vi "WS1050 BURN EFUSE.vi"() -> ()   [LabVIEW 2009]
panel:
  in  "READBACK":bool
  out "error out 2":errorcluster
  out "Fuse Readback":string
  in  "BIT TO BURN":string="07450F"
  in  "stop":bool
  out "VISA resource name out":refnum<visa-resource-name>
  out "error out":errorcluster
  in  "error in (no error)":errorcluster
  in  "VISA resource name":refnum<visa-resource-name>="COM1"
  in  "PUSH BUTTON \nTO START TEST":bool
  # "TEST PROCEDURE TO BURN FUSE T7\n\n1. BIT TO BURN \"ENTER 0745XX\"\n2. INCREASE VDD TO 5V \"JUMPER THE YELLOW WIRE TO 5V\"\n3. DECREASE VDD TO 3.3V THEN MOVE JUMPER TO GND\n4. COMPLETED\n5. READ BACK TO VERIFY FUSE"
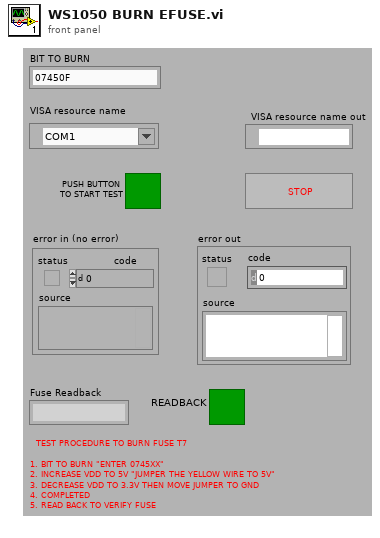
[diagram p1: front panel]
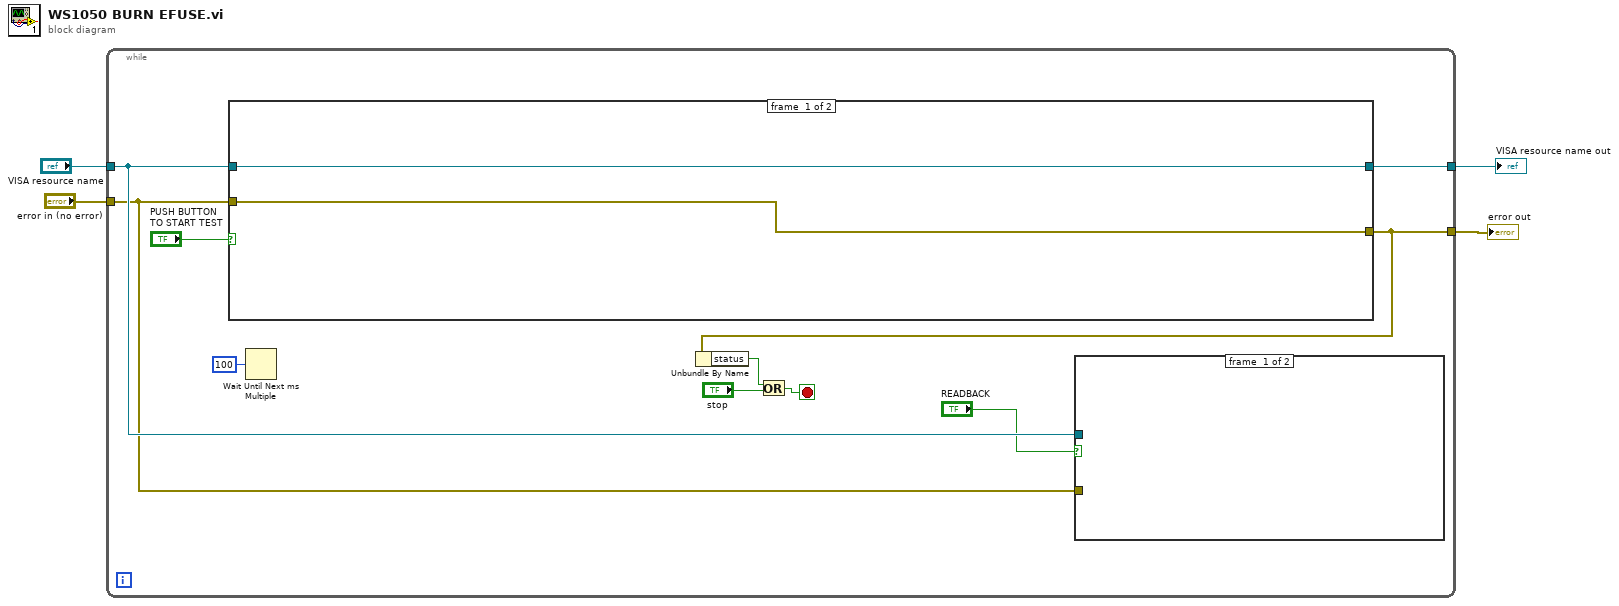
[diagram p0: block diagram]
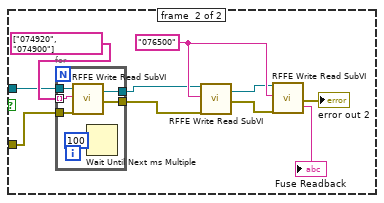
[diagram p2: hidden frame]
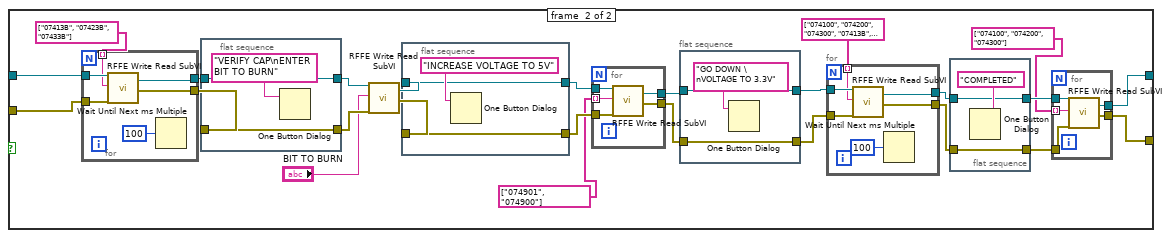
[diagram p3: hidden frame]
diagram:
  n1 = while {
    tunnel: "VISA resource name" -> [w7]
    tunnel: "error in (no error)" -> [w6]
    tunnel: [w11] -> w1
    tunnel: [w13] -> w2
    stop <- w8 stop-if-true
    n2 = case shown="True" "PUSH BUTTON \nTO START TEST" {
      tunnel: w7 -> [w31 w57]
      tunnel: w6 -> [w32 w56]
      tunnel: [w32 w37] -> w11
      tunnel: [w31 w36] -> w13
      frame #0 {
      }
      frame #1 {
        n3 = for {
          tunnel: w57 -> [w91]
          tunnel: w56 -> [w90]
          tunnel: string[] ["07413B", "07423B", "07433B"] -> [w89] mode=indexing
          tunnel: [w87] -> w54
          tunnel: [w86] -> w53
          n4 = call "RFFE Write Read SubVI.vi"("VISA resource name"=w91, "write buffer"=w89, "error in (no error)"=w90) -> ("VISA resource name out"=w86:refnum<visa-resource-name>, "error out"=w87:errorcluster)  [unwired: 12 in, 3 out]
          n5 = Wait Until Next ms Multiple(millisecond multiple=u32 100) -> ()  [unwired: 1 out]
        }
        n6 = flat-sequence {
          tunnel: w54 -> [w84]
          tunnel: [w84] -> w51
          tunnel: w53 -> [w83]
          tunnel: [w83] -> w52
          frame #0 {
            n7 = One Button Dialog(message="VERIFY CAP\nENTER BIT TO BURN") -> ()  [unwired: 1 in, 1 out]
          }
        }
        n8 = call "RFFE Write Read SubVI.vi"("VISA resource name"=w52, "write buffer"="BIT TO BURN", "error in (no error)"=w51) -> ("VISA resource name out"=w49:refnum<visa-resource-name>, "error out"=w48:errorcluster)  [unwired: 12 in, 3 out]
        n9 = flat-sequence {
          tunnel: w48 -> [w81]
          tunnel: [w81] -> w46
          tunnel: w49 -> [w80]
          tunnel: [w80] -> w47
          frame #0 {
            n10 = One Button Dialog(message="INCREASE VOLTAGE TO 5V") -> ()  [unwired: 1 in, 1 out]
          }
        }
        n11 = for {
          tunnel: w47 -> [w79]
          tunnel: w46 -> [w78]
          tunnel: string[] ["074901", "074900"] -> [w77] mode=indexing
          tunnel: [w76] -> w44
          tunnel: [w75] -> w43
          n12 = call "RFFE Write Read SubVI.vi"("VISA resource name"=w79, "write buffer"=w77, "error in (no error)"=w78) -> ("VISA resource name out"=w76:refnum<visa-resource-name>, "error out"=w75:errorcluster)  [unwired: 12 in, 3 out]
        }
        n13 = flat-sequence {
          tunnel: w43 -> [w73]
          tunnel: [w73] -> w33
          tunnel: w44 -> [w72]
          tunnel: [w72] -> w34
          frame #0 {
            n14 = One Button Dialog(message="GO DOWN \nVOLTAGE TO 3.3V") -> ()  [unwired: 1 in, 1 out]
          }
        }
        n15 = for {
          tunnel: w34 -> [w71]
          tunnel: w33 -> [w70]
          tunnel: string[] ["074100", "074200", "074300", "07413B", "07423B", "07433B"] -> [w69] mode=indexing
          tunnel: [w67] -> w40
          tunnel: [w66] -> w41
          n16 = call "RFFE Write Read SubVI.vi"("VISA resource name"=w71, "write buffer"=w69, "error in (no error)"=w70) -> ("VISA resource name out"=w66:refnum<visa-resource-name>, "error out"=w67:errorcluster)  [unwired: 12 in, 3 out]
          n17 = Wait Until Next ms Multiple(millisecond multiple=u32 100) -> ()  [unwired: 1 out]
        }
        n18 = flat-sequence {
          tunnel: w40 -> [w64]
          tunnel: [w64] -> w38
          tunnel: w41 -> [w63]
          tunnel: [w63] -> w39
          frame #0 {
            n19 = One Button Dialog(message="COMPLETED") -> ()  [unwired: 1 in, 1 out]
          }
        }
        n20 = for {
          tunnel: w39 -> [w62]
          tunnel: w38 -> [w61]
          tunnel: [w60] -> w37
          tunnel: [w59] -> w36
          tunnel: string[] ["074100", "074200", "074300"] -> [w58] mode=indexing
          n21 = call "RFFE Write Read SubVI.vi"("VISA resource name"=w62, "write buffer"=w58, "error in (no error)"=w61) -> ("VISA resource name out"=w59:refnum<visa-resource-name>, "error out"=w60:errorcluster)  [unwired: 12 in, 3 out]
        }
      }
    }
    n22 = Wait Until Next ms Multiple(millisecond multiple=u32 100) -> ()  [unwired: 1 out]
    n23 = Unbundle By Name(w11) -> ("status"=w10:bool)
    n24 = Or(x=w10, y="stop") -> (x .or. y?=w8:bool)
    n25 = case shown="True" "READBACK" {
      tunnel: w7 -> [_ w23]
      tunnel: w6 -> [_ w22]
      frame #0 {
      }
      frame #1 {
        w20 = "076500" ("write buffer")
        n26 = for {
          tunnel: w23 -> [w30]
          tunnel: w22 -> [w29]
          tunnel: string[] ["074920", "074900"] -> [w27] mode=indexing
          tunnel: [w26] -> w16
          tunnel: [w25] -> w17
          n27 = call "RFFE Write Read SubVI.vi"("VISA resource name"=w30, "write buffer"=w27, "error in (no error)"=w29) -> ("VISA resource name out"=w25:refnum<visa-resource-name>, "error out"=w26:errorcluster)  [unwired: 12 in, 3 out]
          n28 = Wait Until Next ms Multiple(millisecond multiple=u32 100) -> ()  [unwired: 1 out]
        }
        n29 = call "RFFE Write Read SubVI.vi"("VISA resource name"=w17, "write buffer"=w20, "error in (no error)"=w16) -> ("VISA resource name out"=w19:refnum<visa-resource-name>, "error out"=w18:errorcluster)  [unwired: 12 in, 3 out]
        n30 = call "RFFE Write Read SubVI.vi"("VISA resource name"=w19, "write buffer"=w20, "error in (no error)"=w18) -> ("Fuse Readback"=→"Fuse Readback":string, "error out"=→"error out 2":errorcluster)  [unwired: 12 in, 3 out]
      }
    }
  }
  "error out" <- w1
  "VISA resource name out" <- w2
